vi "EMV PI Controller Estimate.vi"(6 "User Setpoint Temperature":u16, 8 "error in (no error)":errorcluster, 11 "T6 Temp":dbl=140.0) -> (0 "error out":errorcluster)   [LabVIEW 2016]
panel:
  out "PI Flow Dectection":bool
  out "Current T6 Temperatures":dbl[](array[numeric])
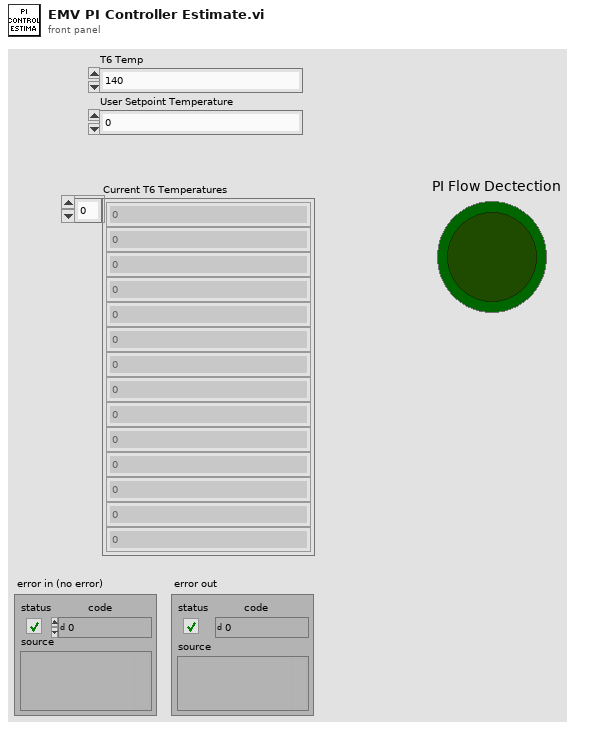
[diagram p1: front panel]
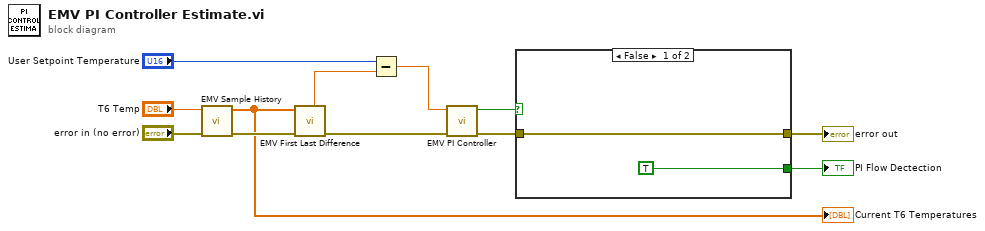
[diagram p0: block diagram]
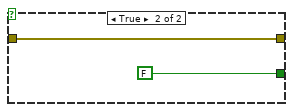
[diagram p2: hidden frame]
diagram:
  n1 = call "EMV Sample History.vi"("error in (no error)"="error in (no error)", "T6 Temp"="T6 Temp") -> ("error out"=w3:errorcluster, "T6 History"=w1:dbl[])  [unwired: 8 in]
  "Current T6 Temperatures" <- w1
  n2 = call "EMV First Last Difference.vi"("error in (no error)"=w3, "Current T6 Temperatures in"=w1) -> ("error out"=w10:errorcluster, "Current Temperature"=w12:dbl)  [unwired: 5 in, 3 out]
  n3 = Subtract(x="User Setpoint Temperature", y=w12) -> (x-y=w5:dbl)
  n4 = call "EMV PI Controller.vi"("error in (no error)"=w10, "Error"=w5) -> ("error out"=w7:errorcluster, "PI Saturated"=w9:bool)  [unwired: 8 in]
  n5 = case shown="False" w9 {
    tunnel: [TRUE FALSE] -> w8
    tunnel: w7 -> [w13 w15]
    tunnel: [w13 w15] -> w6
    frame False {
    }
    frame True {
    }
  }
  "error out" <- w6
  "PI Flow Dectection" <- w8
